vi "Initialization VI.vi"(8 "error in (no error)":errorcluster, 10 "Custom XML":string, 11 "Device Item Ref in":T1 format="%.0x") -> (0 "error out":errorcluster, 3 "Device Item Ref out":T1 format="%.0x")   [LabVIEW 2019, in "Instrument Addon System Explorer.lvlib"]
uses:
  Instrument Addon System Explorer.lvlib
  <vilib>/NI VeriStand/Custom Device API/Custom Device Item Ref.ctl
  Addon Shared/Types/FG Control.ctl
  Addon Shared/SubVIs/Constants.vi
  <vilib>/NI/NI VeriStand Advanced SysDef API/SysDef API/SysDef.Property.Get.vi
  <vilib>/NI/NI VeriStand Advanced SysDef API/_SubVIs/SysDef.Property.Get.String.vi
  <vilib>/NI/NI VeriStand Advanced SysDef API/SysDef API/SysDef.Property.Set.vi
  <vilib>/NI/NI VeriStand Advanced SysDef API/_SubVIs/SysDef.Property.Set.String.vi
  Addon Shared/Instrument Addon Shared.lvlib
  <vilib>/NI VeriStand/Custom Device API/Custom Device API.lvlib
  <vilib>/NI/NI VeriStand Custom Device Import and Export Tool/ImportExport.lvlib
  APIs/Scripting API/Instrument Addon Scripting API.lvlib
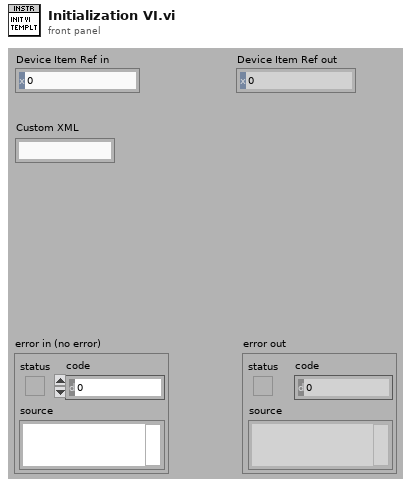
[diagram p1: front panel]
types:
  T1 = typedef "Custom Device API.lvlib/Custom Device Item Ref.ctl" = u64
  T2 = typedef "Instrument Addon Shared.lvlib/FG Control.ctl" = enum16{"Get", "Set"}
  T3 = typedef "Instrument Addon System Explorer.lvlib/Initial User Selection.ctl" = cluster{"Protocol":string}
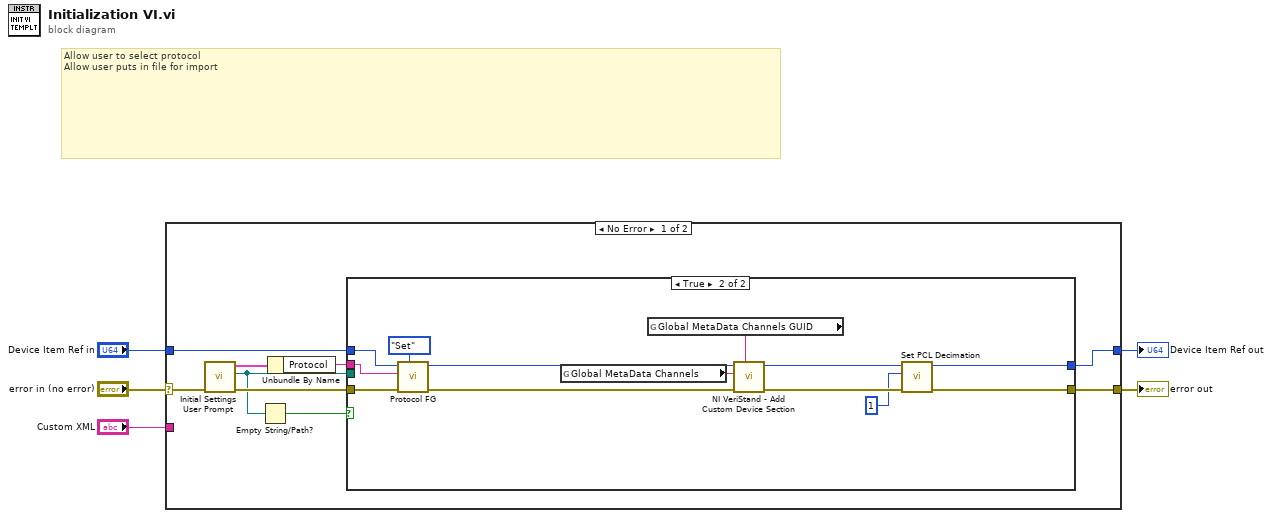
[diagram p0: block diagram]
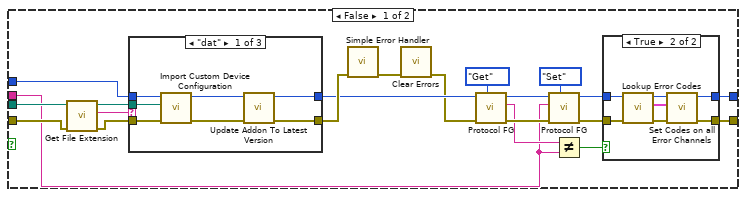
[diagram p2: hidden frame]
diagram:
  # "Allow user to select protocol\nAllow user puts in file for import"
  n1 = case shown="No Error" "error in (no error)" {
    selector: "error in (no error)" -> [w14 w69]
    tunnel: [w12 w69] -> w5
    tunnel: [w8 w68] -> w3
    tunnel: "Device Item Ref in" -> [w9 w68]
    tunnel: "Custom XML" -> [_ _]
    frame No Error {
      n2 = call "Initial Settings User Prompt.vi"("error in (no error)"=w14) -> ("error out"=w13:errorcluster, "Path out"=w6:path, "Initial Settings"=w11:T3)  [unwired: 8 in]
      n3 = Empty String/Path?(string/path=w6) -> (empty?=w7:bool)
      n4 = Unbundle By Name(w11) -> ("Protocol"=w10:string)
      n5 = case shown="True" w7 {
        tunnel: w13 -> [w29 w67]
        tunnel: [w25 w59] -> w12
        tunnel: w10 -> [w16 w61]
        tunnel: w9 -> [w35 w66]
        tunnel: [w23 w57] -> w8
        tunnel: w6 -> [w31 _]
        frame False {
          n6 = call <vilib>:"Get File Extension.vi"("error in (no error)"=w29, "file"=w31) -> ("error out"=w28:errorcluster, "lowercase file extension"=w27:string, "dup file"=w30:path)  [unwired: 5 in, 2 out]
          n7 = case shown="\"dat\"" w27 {
            tunnel: w28 -> [w51 w53 w54]
            tunnel: w35 -> [w50 w52 w55]
            tunnel: w30 -> [w49 _ _]
            tunnel: [w45 w52 w55] -> w21
            tunnel: [w47 w53 w54] -> w32
            frame "dat" {
              n8 = call <vilib>:"Import Custom Device Configuration.vi"("error in (no error)"=w51, "Path"=w49, "NodeID"=w50) -> ("error out"=w48:errorcluster, "NodeID out"=w46:u64)  [unwired: 6 in, 1 out]
              n9 = call "Update Addon To Latest Version.vi"("error in (no error)"=w48, "Device Item Ref in"=w46) -> ("error out"=w47:errorcluster, "Device Item Ref out"=w45:T1)  [unwired: 8 in]
            }
            frame "xml" {
            }
            frame Default {
            }
          }
          n10 = call <vilib>:"Simple Error Handler.vi"("error in (no error)"=w32) -> ("error out"=w33:errorcluster)  [unwired: 4 in, 4 out]
          n11 = call <vilib>:"Clear Errors.vi"("error in (no error)"=w33) -> ("error out"=w18:errorcluster)  [unwired: 5 in, 1 out]
          n12 = call "Protocol FG.vi"("Action"=FG_Control."Get", "error in (no error)"=w18, "Device Item Ref in"=w21) -> ("error out"=w19:errorcluster, "Protocol out"=w17:string, "Item Ref out"=w20:T1)  [unwired: 6 in]
          n13 = call "Protocol FG.vi"("Action"=FG_Control."Set", "error in (no error)"=w19, "Protocol"=w16, "Device Item Ref in"=w20) -> ("error out"=w26:errorcluster, "Item Ref out"=w24:T1)  [unwired: 5 in, 1 out]
          n14 = Not Equal?(x=w17, y=w16) -> (x != y?=w15:bool)
          n15 = case shown="True" w15 {
            tunnel: w26 -> [w37 w41]
            tunnel: [w37 w40] -> w25
            tunnel: w24 -> [w36 w39]
            tunnel: [w36 w38] -> w23
            frame False {
            }
            frame True {
              n16 = call "Lookup Error Codes.vi"("error in (no error)"=w41, "Node Ptr"=w39) -> ("error out"=w43:errorcluster, "Error Codes"=w42:cluster{"Code":i32, "String":string}[], "Node Ptr out"=w44:u64)  [unwired: 7 in]
              n17 = call "Set Codes on all Error Channels.vi"("error in (no error)"=w43, "Error Codes"=w42, "Node Ptr in"=w44) -> ("error out"=w40:errorcluster, "Section Ref out"=w38:T1)  [unwired: 7 in]
            }
          }
        }
        frame True {
          n18 = call "Protocol FG.vi"("Action"=FG_Control."Set", "error in (no error)"=w67, "Protocol"=w61, "Device Item Ref in"=w66) -> ("error out"=w60:errorcluster, "Item Ref out"=w65:T1)  [unwired: 5 in, 1 out]
          n19 = global read "Constants.vi" "Global MetaData Channels"() -> (w62:string)
          n20 = global read "Constants.vi" "Global MetaData Channels GUID"() -> (w63:string)
          n21 = call <vilib>:"NI VeriStand - Add Custom Device Section.vi"("GUID (Default Section)"=w63, "Section Name"=w62, "Parent Ref in"=w65) -> ("Parent Ref out"=w58:T1)  [unwired: 5 in, 3 out]
          n22 = call "Set PCL Decimation.vi"("error in (no error)"=w60, "PCL decimation"=u32 1, "instrument addon refnum in"=w58) -> ("error out"=w59:errorcluster, "instrument addon refnum"=w57:T1)  [unwired: 7 in]
        }
      }
    }
    frame Error {
    }
  }
  "error out" <- w5
  "Device Item Ref out" <- w3
